vi "FGV_GOpark.vi"(8 "errin":errorcluster) -> (0 "errout":errorcluster)   [LabVIEW 2020]
uses:
  02 SLIM ZEN WS 500/SubVi/FGV.ctl
  02 SLIM ZEN WS 500/SubVi/VG CAN VEH ON.vi
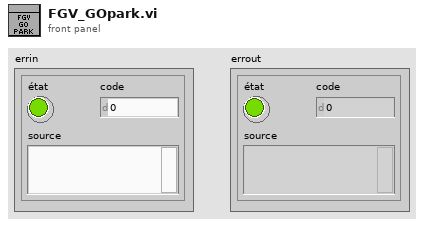
[diagram p1: front panel]
types:
  T1 = typedef "FGV.ctl" = enum16{"GET", "SET", "RAZ"}
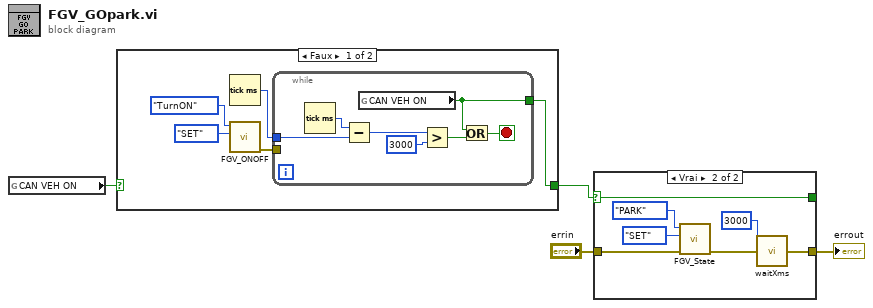
[diagram p0: block diagram]
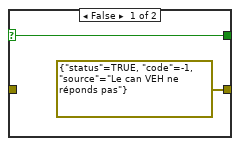
[diagram p2: hidden frame]
diagram:
  n1 = global read "VG CAN VEH ON.vi" "CAN VEH ON"() -> (w4:bool)
  n2 = case shown="Faux" w4 {
    selector: w4 -> [_ w17]
    tunnel: [w6 w17] -> w3
    frame False {
      n3 = Tick Count (ms)() -> (millisecond timer value=w7:u32)
      n4 = call "FGV_ONOFF.vi"("CMD"=FGV."SET", "ONOFF"=enum16{"TurnON", "TurnOFF"}."TurnON") -> ("errout"=w5:errorcluster)  [unwired: 8 in, 1 out]
      n5 = while {
        tunnel: w7 -> [w15]
        tunnel: [w10] -> w6
        tunnel: w5 -> [_]
        stop <- w12 stop-if-true
        n6 = Tick Count (ms)() -> (millisecond timer value=w16:u32)
        n7 = Subtract(x=w16, y=w15) -> (x-y=w14:u32)
        n8 = global read "VG CAN VEH ON.vi" "CAN VEH ON"() -> (w10:bool)
        n9 = Greater?(x=w14, y=u32 3000) -> (0:w11:bool)
        n10 = Or(x=w10, y=w11) -> (x .or. y?=w12:bool)
      }
    }
    frame True {
    }
  }
  n11 = case shown="Vrai" w3 {
    selector: w3 -> [w19 w21]
    tunnel: [errorcluster {"status"=TRUE, "code"=-1, "source"="Le can VEH ne réponds pas"} ("errout") w23] -> w2
    tunnel: [w19 w21] -> _
    tunnel: "errin" -> [_ w20]
    frame False {
    }
    frame True {
      n12 = call "FGV_State.vi"("errin"=w20, "CMD"=FGV."SET" ("Énum"), "State"=enum16{"OFF", "PARK", "DRIVE", "LOAD"}."PARK") -> ("errout"=w24:errorcluster)  [unwired: 7 in, 1 out]
      n13 = call "waitXms.vi"("attente (ms)"=u32 3000, "errin"=w24) -> ("errout"=w23:errorcluster)  [unwired: 13 in]
    }
  }
  "errout" <- w2
